vi "pcap-finddev.vi"() -> (0 "String 4":string, 1 "String 3":string, 2 "String 2":string, 3 "String":string, 4 "String 5":string)   [LabVIEW 2017]
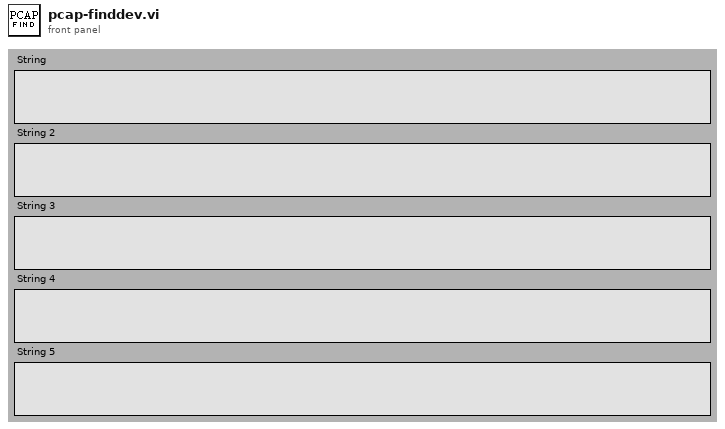
[diagram p1: front panel]
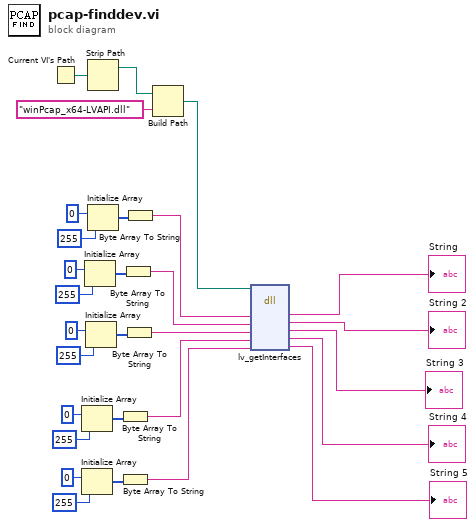
[diagram p0: block diagram]
diagram:
  n1 = Current VI's Path() -> (path=w4:path)
  n2 = Initialize Array(u8 0, 255) -> (w13:u8[])
  n3 = Initialize Array(u8 0, 255) -> (w10:u8[])
  n4 = Initialize Array(u8 0, 255) -> (w19:u8[])
  n5 = Initialize Array(u8 0, 255) -> (w16:u8[])
  n6 = Strip Path(path=w4) -> (stripped path=w3:path)  [unwired: 1 out]
  n7 = Initialize Array(u8 0, 255) -> (w22:u8[])
  n8 = Byte Array To String(unsigned byte array=w13) -> (string=w6:string)
  n9 = Byte Array To String(unsigned byte array=w10) -> (string=w5:string)
  n10 = Byte Array To String(unsigned byte array=w19) -> (string=w8:string)
  n11 = Byte Array To String(unsigned byte array=w16) -> (string=w7:string)
  n12 = Byte Array To String(unsigned byte array=w22) -> (string=w9:string)
  n13 = Build Path(base path=w3, name or relative path="winPcap_x64-LVAPI.dll") -> (appended path=w1:path)
  n14 = dll-call lib="C:/Users/ucbtspu.AD/OneDrive - University College London/Local SCC/SilverLab-Microscope x64/Ethernet/winPcap_x64-LVAPI.dll" fn="lv_getInterfaces"(path in=w1, w9, w8, w7, w6, w5) -> (→"String":string, →"String 2":string, →"String 3":string, →"String 4":string, →"String 5":string)  [unwired: 3 in, 2 out]
